vi "Initialize and Run FPGA VI.vi"(7 "resource name":T1, 8 "error in (no error)":errorcluster, 10 "Timeout Period (ticks)":u64, 11 "Control Period (ticks)":u32) -> (0 "error out":errorcluster, 3 "FPGA VI Reference Out":T2)   [LabVIEW 2013]
uses:
  controls/FPGA VI Reference.ctl
  <vilib>/userdefined/High Color/nirio_resource_hc.ctl
  <vilib>/FPGAPlugInAG/cRIO-9075/niLvFpga_Open_cRIO-9075.vi
  <vilib>/FPGAPlugInAG/cRIO-9075/niLvFpga_Reset_cRIO-9075.vi
  <vilib>/Utility/error.llb/Error Cluster From Error Code.vi
  <vilib>/rvi/errors/niLvFpgaAdjustHostInterfaceError.vi
  <vilib>/FPGAPlugInAG/cRIO-9075/niLvFpga_Run_cRIO-9075.vi
  <vilib>/rvi/interface/nirviOpenFPGA/nirviOpenFPGA.xnode
  FPGA Bitfiles/crio-FPGA-contro_FPGATarget_FPGAMain_4HKUk4gb9wY.lvbitx
  <vilib>/rvi/interface/nirviMethod/nirviMethod.xnode
  <vilib>/rvi/interface/nirviReadWriteControl/nirviReadWriteControl.xnode
  NiFpgaLv.dll
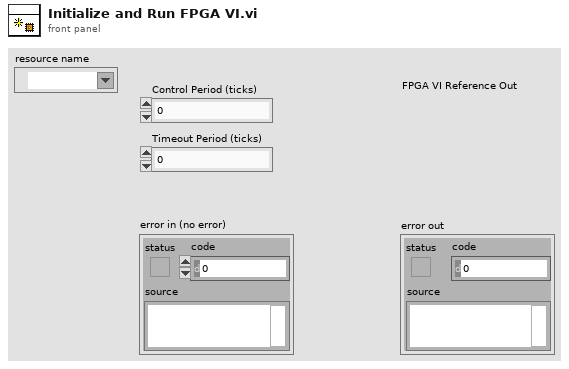
[diagram p1: front panel]
types:
  T1 = typedef "nirio_resource_hc.ctl" = tag
  T2 = typedef "FPGA VI Reference.ctl" = refnum<k20>
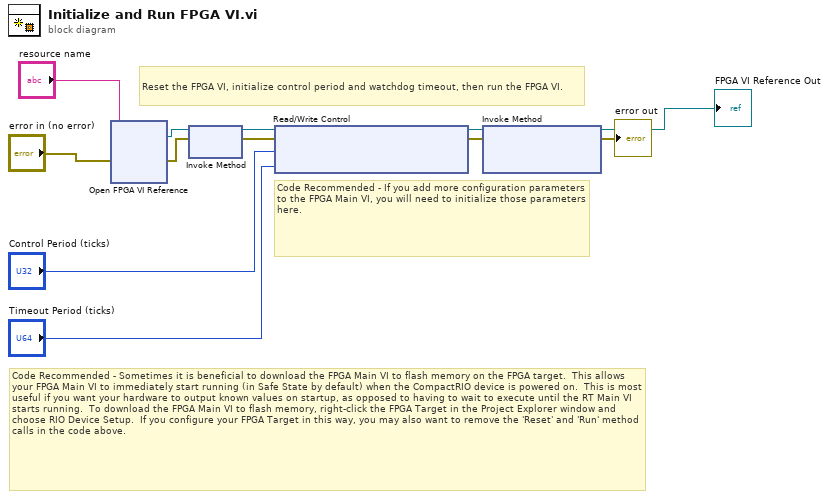
[diagram p0: block diagram]
diagram:
  # "Code Recommended - Sometimes it is beneficial to download the FPGA Main VI to flash memory on the FPGA target.  This allows your FPGA Main VI to immediately start running (in Safe State by default) when the CompactRIO device is powered on.  This is most useful if you want your hardware to output known values on startup, as opposed to having to wait to execute until the RT Main VI starts running.  To download the FPGA Main VI to flash memory, right-click the FPGA Target in the Project Explorer window and choose RIO Device Setup.  If you configure your FPGA Target in this way, you may also want to remove the 'Reset' and 'Run' method calls in the code above."
  # "Reset the FPGA VI, initialize control period and watchdog timeout, then run the FPGA VI."
  # "Code Recommended - If you add more configuration parameters to the FPGA Main VI, you will need to initialize those parameters here."
  n1 = xnode "Open FPGA VI Reference"("error in"="error in (no error)", "resource name"="resource name") -> ("FPGA VI Reference Out"=w4:T2, "error out"=w5:errorcluster)
  n2 = xnode "Invoke Method"("FPGA VI Reference In"=w4, "error in"=w5) -> ("FPGA VI Reference Out"=w3:T2, "error out"=w6:errorcluster)
  n3 = xnode "Read/Write Control"("FPGA VI Reference In"=w3, "error in"=w6, "Control Period (ticks)"="Control Period (ticks)", "Watchdog Timeout Period (ticks)"="Timeout Period (ticks)") -> ("FPGA VI Reference Out"=w8:T2, "error out"=w9:errorcluster)
  n4 = xnode "Invoke Method"("FPGA VI Reference In"=w8, "error in"=w9) -> ("FPGA VI Reference Out"=→"FPGA VI Reference Out":T2, "error out"=→"error out":errorcluster)  [unwired: 1 in]
